vi "RSD Command Send.vi"(0 "VISA resource name":refnum<visa-resource-name>, 1 "Checksum used":bool=TRUE, 5 "Address":u8, 7 "Count number":u8, 9 "D-register number":u8, 11 "error in (no error)":errorcluster) -> (4 "VISA resource name out":refnum<visa-resource-name>, 6 "Request":string, 15 "error out":errorcluster)   [LabVIEW 2017, in "Samwontech TEMP2xxx.lvlib"]
doc: "RSD Command is used to read data in a part of D-Regiater by consecutive address in sequence"
uses:
  <instrlib>/Samwontech TEMP2xxx/Samwontech TEMP2xxx.lvlib
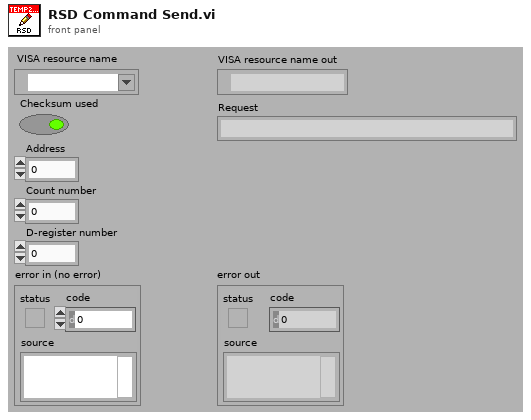
[diagram p1: front panel]
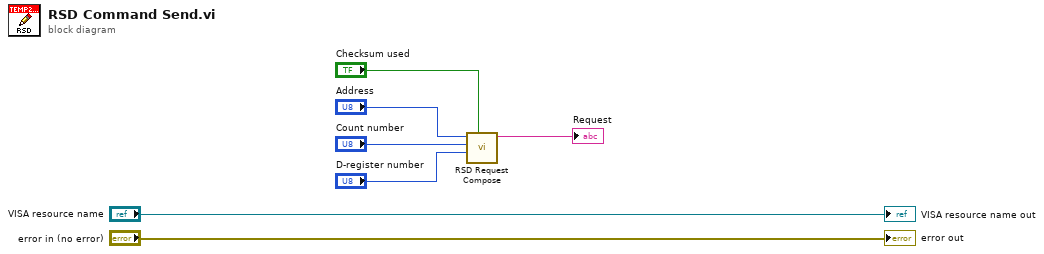
[diagram p0: block diagram]
diagram:
  n1 = call <instrlib>:"RSD Request Compose.vi"("Checksum used"="Checksum used", "D-register number"="D-register number", "Count number"="Count number", "Address"="Address") -> ("Request"=→"Request":string)  [unwired: 7 in]
  "error out" <- "error in (no error)"
  "VISA resource name out" <- "VISA resource name"
